vi "Auto Intake&Lift.vi"(8 "armsClose":bool, 9 "Switch/Scale?":bool, 10 "intakeSpeed":dbl, 11 "elevatorSpeed":dbl) -> ()   [LabVIEW 2017]
uses:
  Common Code/Intake And Elevator States.ctl
  Common Code/Elevator Mode.ctl
  Common Code/Intake Mode.ctl
  Common Code/Elevator State.ctl
  Robot Global Data.vi
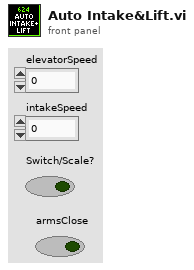
[diagram p1: front panel]
types:
  T1 = typedef "Intake Mode.ctl" = enum16{"Auto", "Semi Auto", "Manual"}
  T2 = typedef "Elevator Mode.ctl" = enum16{"Semi Auto", "Manual", "Auto"}
  T3 = typedef "Intake And Elevator States.ctl" = enum16{"Idle", "Pick Up Cube", "Switch", "Scale ", "Endgame"}
  T4 = typedef "Intake And Elevator Command Cluster.ctl" = cluster{"States ":T3, "Grab?":bool, "Drop?":bool, "Mode":T5, "Override Lift":bool, "Override Lift":dbl, "High?":bool}
  T5 = typedef "Intake and Elevator Mode.ctl" = enum16{"Auto", "Not Auto"}
  T6 = typedef "Elevator Command Cluster.ctl" = cluster{"Elevator Mode":T2, "Elevator State":T7, "Manual Speed":dbl, "Reset Encoders":bool, "High?":bool}
  T7 = typedef "Elevator State.ctl" = enum16{"Idle", "Ground", "Mid", "Scale", "Switch"}
  T8 = typedef "Intake Command Cluster.ctl" = cluster{"Intake Mode":T1, "Intake States":T9, "Manual Roller Power":dbl, "Manual Close?":bool, "Manual Lift Power":dbl, "Override Lift?":bool, "Override Angle":dbl}
  T9 = typedef "Intake States.ctl" = enum16{"Curl Up", "Override Angle", "Idle", "Drop Mid", "Drop Low", "Outtake", "Intake"}
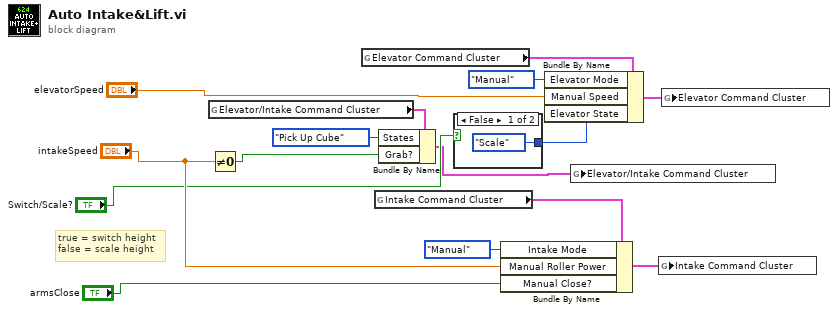
[diagram p0: block diagram]
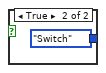
[diagram p2: hidden frame]
diagram:
  # "true = switch height\nfalse = scale height"
  n1 = global read "Robot Global Data.vi" "Elevator/Intake Command Cluster"() -> (w15:T4)
  n2 = Not Equal To 0?(x="intakeSpeed") -> (x != 0?=w13:bool)
  n3 = global read "Robot Global Data.vi" "Elevator Command Cluster"() -> (w12:T6)
  n4 = global read "Robot Global Data.vi" "Intake Command Cluster"() -> (w11:T8)
  n5 = Bundle By Name(cluster=w15, "States"=Intake_And_Elevator_States."Pick Up Cube", "Grab?"=w13) -> (w1:T4)
  n6 = case shown="False" "Switch/Scale?" {
    tunnel: [Elevator_State."Scale" ("Elevator State") Elevator_State."Switch" ("Elevator State")] -> w6
    frame False {
    }
    frame True {
    }
  }
  n7 = Bundle By Name(cluster=w11, "Intake Mode"=Intake_Mode."Manual", "Manual Roller Power"="intakeSpeed", "Manual Close?"="armsClose") -> (w2:T8)
  n8 = Bundle By Name(cluster=w12, "Elevator Mode"=Elevator_Mode."Manual", "Manual Speed"="elevatorSpeed", "Elevator State"=w6) -> (w3:T6)
  n9 = global write "Robot Global Data.vi" "Elevator/Intake Command Cluster"(w1) -> ()
  n10 = global write "Robot Global Data.vi" "Intake Command Cluster"(w2) -> ()
  n11 = global write "Robot Global Data.vi" "Elevator Command Cluster"(w3) -> ()
